vi "MergeFiles.vi"(8 "输出结果":refnum<vi>, 9 "SelectedFormat":refnum<vi>, 10 "FileList":refnum<vi>, 11 "FilesArry":refnum<vi>) -> (2 "Path":path)   [LabVIEW 2015]
panel:
  out "Arry 2":path[](array[path])
  out "第二个子数组":string[](array[string])
  out "Value":string[][](array[string])
  out "Arry1":path[](array[path])
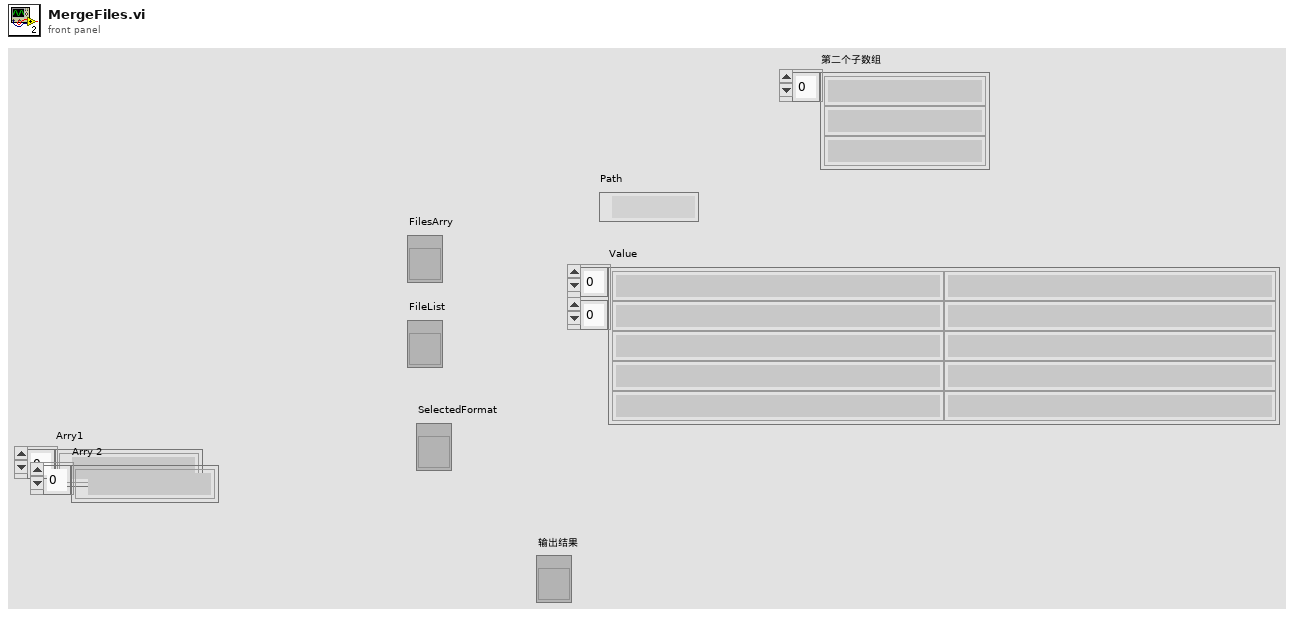
[diagram p1: front panel]
types:
  T1 = enum16{"big-endian, network order", "native, host order", "little-endian"}
  T2 = enum16{"open", "replace", "create", "open or create", "replace or create", "replace or create with confirmation"}
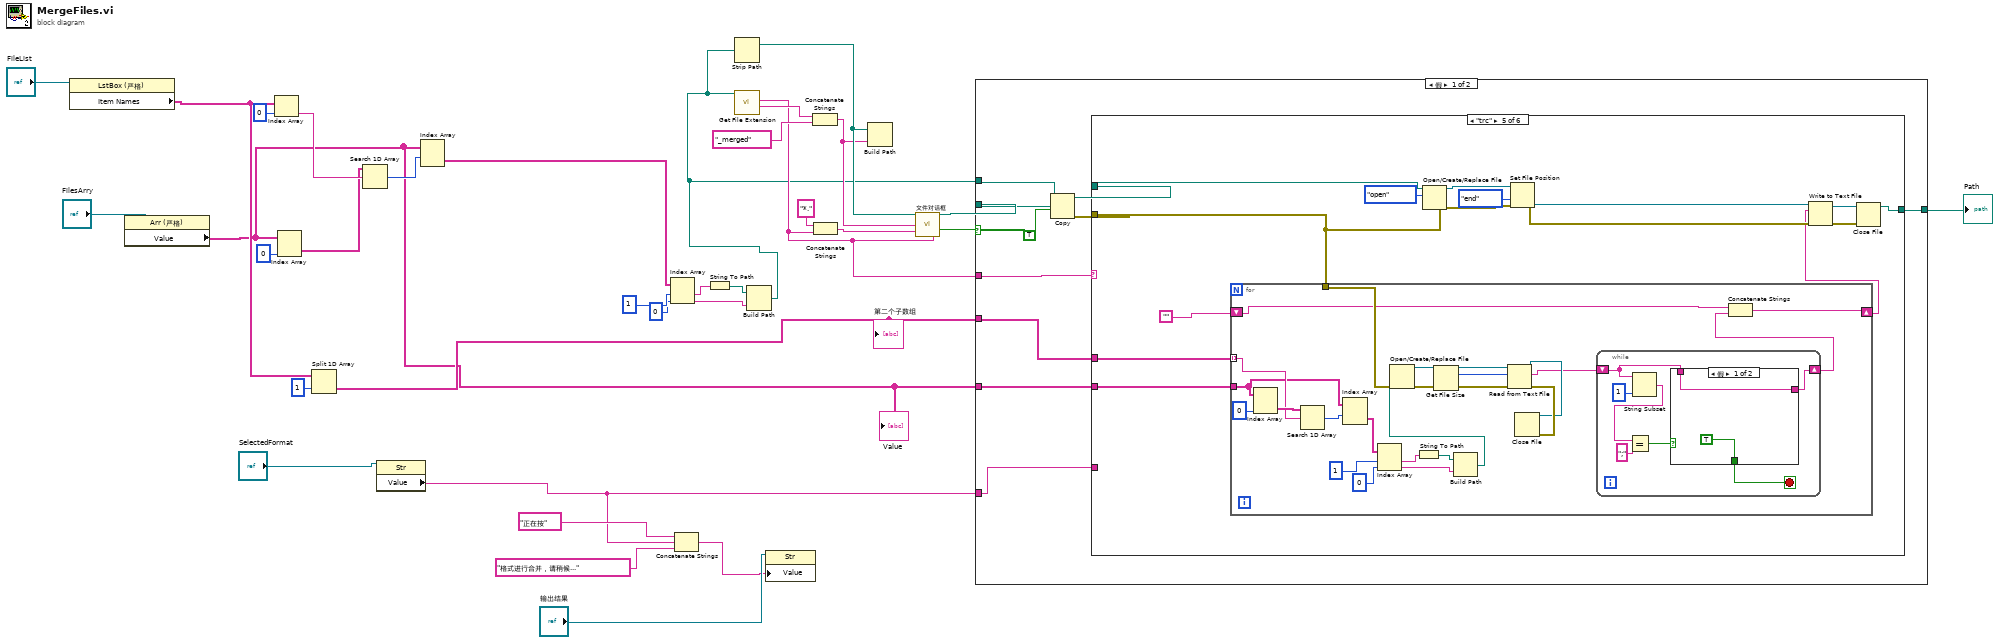
[diagram p0: block diagram]
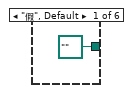
[diagram p2: hidden frame]
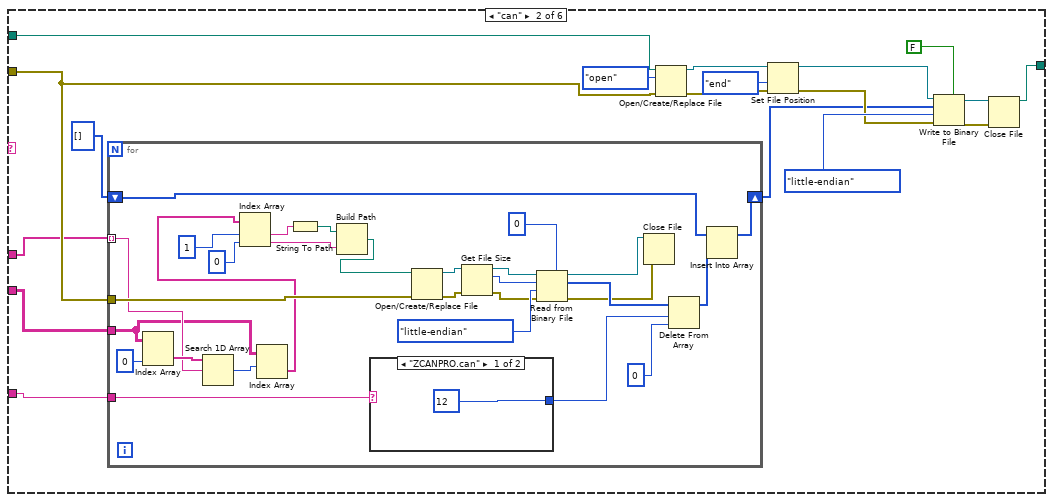
[diagram p3: hidden frame]
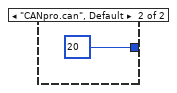
[diagram p4: hidden frame]
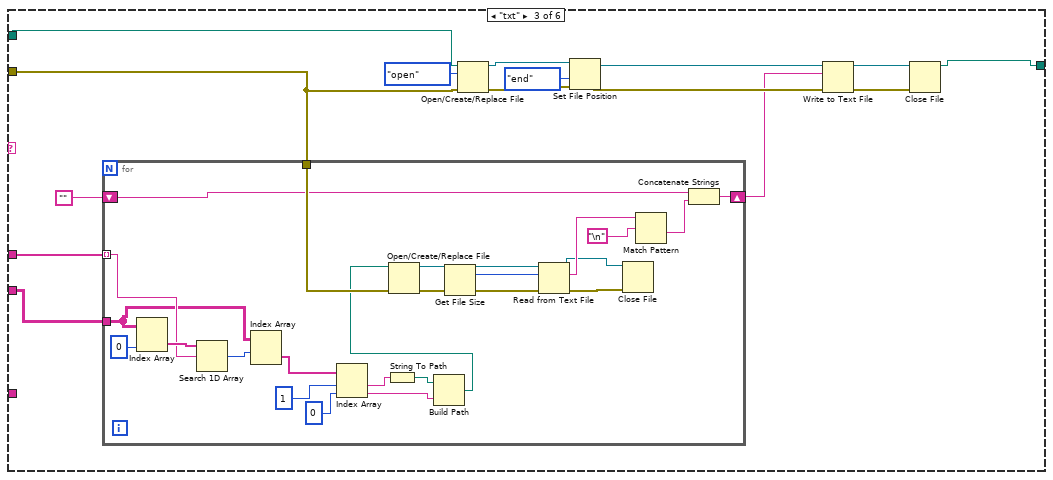
[diagram p5: hidden frame]
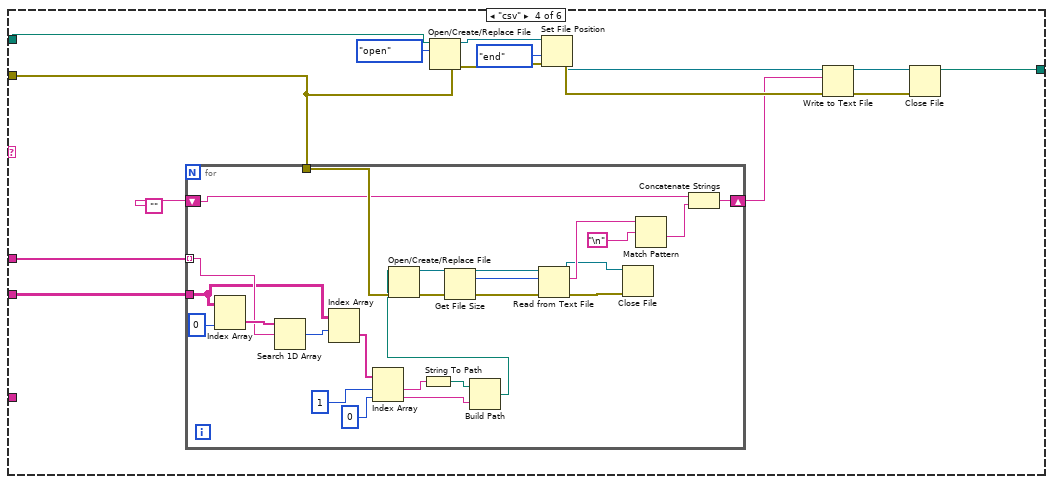
[diagram p6: hidden frame]
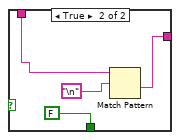
[diagram p7: hidden frame]
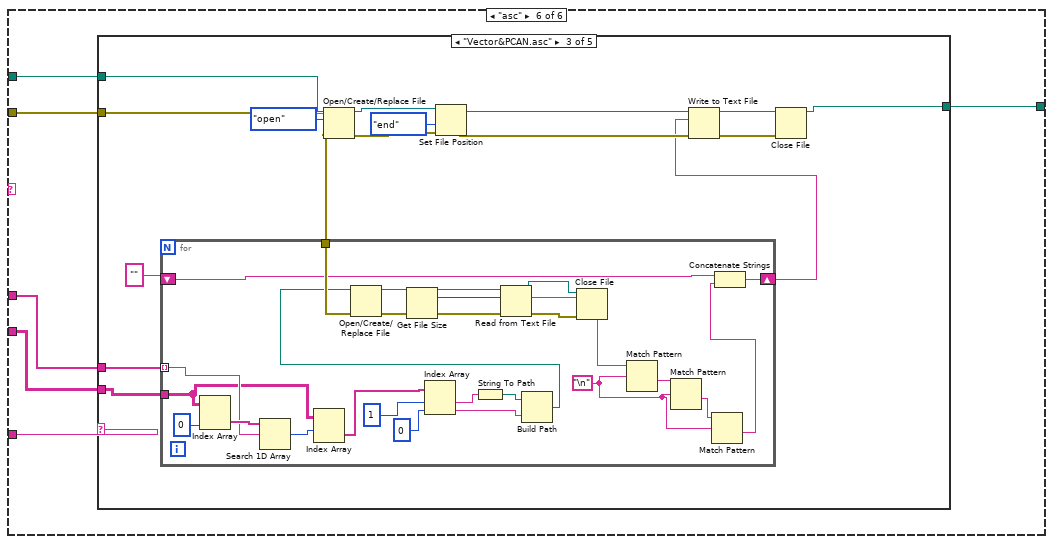
[diagram p8: hidden frame]
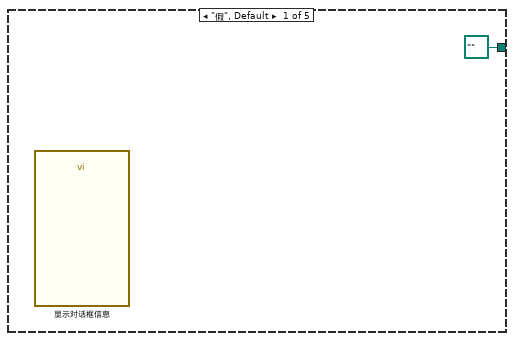
[diagram p9: hidden frame]
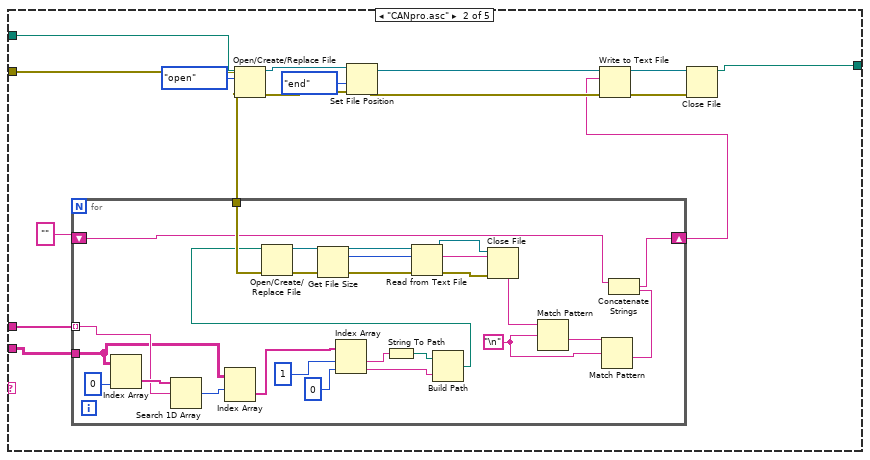
[diagram p10: hidden frame]
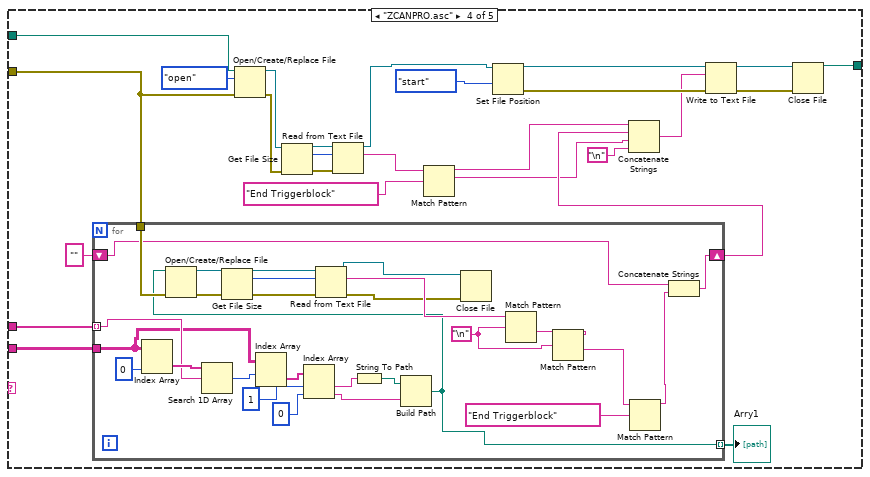
[diagram p11: hidden frame]
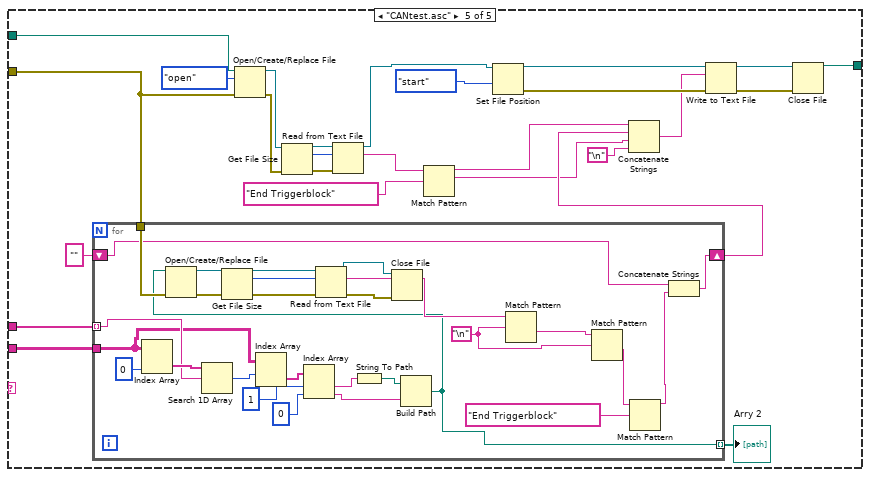
[diagram p12: hidden frame]
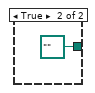
[diagram p13: hidden frame]
diagram:
  n1 = property class="LstBox (严格)"(reference="FileList") -> ("Item Names"=w10:string[])  [unwired: 1 in, 2 out]
  n2 = property class="Arr (严格)"(reference="FilesArry") -> ("Value"=w7:string[][])  [unwired: 1 in, 2 out]
  "Value" <- w7
  n3 = Index Array(array=w10, index=0 ("索引")) -> (element=w14:string)
  n4 = Index Array(array=w7, index (col)=0 ("禁用的索引 (列)")) -> (element=w13:string[])  [unwired: 1 in]
  n5 = Split 1D Array(array=w10, index=1 ("索引")) -> (second subarray=w8:string[])  [unwired: 1 out]
  "第二个子数组" <- w8
  n6 = Search 1D Array(1D array=w13, element=w14) -> (index of element=w12:i32)  [unwired: 1 in]
  n7 = property class="Str"(reference="SelectedFormat") -> ("Value"=w3:string)  [unwired: 1 in, 2 out]
  n8 = Index Array(array=w7, index (row)=w12) -> (element=w11:string[])  [unwired: 1 in]
  n9 = Index Array(array=w11, index #1=1 ("索引"), index #2=0 ("索引")) -> (element #1=w20:string, element #2=w18:string)
  n10 = Concatenate Strings("正在按", w3, "格式进行合并，请稍候...") -> (w1:string)
  n11 = String To Path(string=w20) -> (path=w19:path)
  n12 = Build Path(base path=w19, name or relative path=w18) -> (appended path=w17:path)
  n13 = Strip Path(path=w17) -> (stripped path=w30:path)  [unwired: 1 out]
  n14 = call <vilib>:"Get File Extension.vi"("file"=w17) -> ("filename without extension"=w27:string, "lowercase file extension"=w23:string)  [unwired: 6 in, 3 out]
  n15 = property class="Str"(reference="输出结果", "Value"=w1) -> ()  [unwired: 1 in, 2 out]
  n16 = Concatenate Strings(w27, "_merged" ("字符串")) -> (w29:string)
  n17 = Concatenate Strings("*.", w23) -> (w26:string)
  n18 = Build Path(base path=w30, name or relative path=w29) -> ()  [unwired: 1 out]
  n19 = call "文件对话框"("start path"=w30, "default name"=w29, "pattern (all files)"=w26, "pattern label"=w23) -> ("selected path"=w28:path, "cancelled"=w24:bool)  [unwired: 8 in, 2 out]
  n20 = case shown="假" w24 {
    tunnel: w28 -> [w44 _]
    tunnel: w17 -> [w42 _]
    tunnel: w23 -> [w39 _]
    tunnel: w3 -> [w38 _]
    tunnel: w8 -> [w37 _]
    tunnel: w7 -> [w36 _]
    tunnel: [w35 path "" ("path")] -> w6
    frame False {
      n21 = Copy(9:TRUE, 10:w44, 11:w42) -> (0:w40:errorcluster, 3:w43:path)  [unwired: 2 in, 1 out]
      n22 = case shown="\"trc\"" w39 {
        tunnel: w43 -> [_ w62 w108 w148 w188 w232]
        tunnel: w40 -> [_ w53 w104 w144 w184 w231]
        tunnel: w38 -> [_ w52 _ _ _ w230]
        tunnel: w37 -> [_ w49 w98 w138 w178 w229]
        tunnel: w36 -> [_ w47 w96 w136 w176 w228]
        tunnel: [path "" ("path") w46 w95 w135 w175 w227] -> w35
        frame "假", Default {
        }
        frame "can" {
          n23 = for {
            tunnel: w53 -> [w82]
            tunnel: w52 -> [w81]
            tunnel: w49 -> [w67] mode=indexing
            shift-right: [w71] -> w54
            shift-left: u8[] [] -> [w70]
            tunnel: w47 -> [w66]
            n24 = Index Array(array=w66, index (col)=0 ("禁用的索引 (列)")) -> (element=w69:string[])  [unwired: 1 in]
            n25 = Search 1D Array(1D array=w69, element=w67) -> (index of element=w68:i32)  [unwired: 1 in]
            n26 = Index Array(array=w66, index (row)=w68) -> (element=w65:string[])  [unwired: 1 in]
            n27 = Index Array(array=w65, index #1=1 ("索引"), index #2=0 ("索引")) -> (element #1=w74:string, element #2=w78:string)
            n28 = String To Path(string=w74) -> (path=w75:path)
            n29 = Build Path(base path=w75, name or relative path=w78) -> (appended path=w73:path)
            n30 = case shown="\"ZCANPRO.can\"" w81 {
              tunnel: [12 ("长度") 20 ("长度")] -> w84
              frame "ZCANPRO.can" {
              }
              frame "CANpro.can", Default {
              }
            }
            n31 = Open/Create/Replace File(file path (use dialog)=w73, error in=w82) -> (refnum out=w91:refnum<file>, error out=w90:errorcluster)  [unwired: 4 in, 1 out]
            n32 = Get File Size(file=w91, error in=w90) -> (refnum out=w89:refnum<file>, size (in bytes)=w88:i64, 0:w87:errorcluster)
            n33 = Read from Binary File(5:u8 0, 8:w87, 9:T1."little-endian" ("字节顺序(0:big-endian, network order)"), 10:w88, 11:w89) -> (0:w79:errorcluster, 2:w83:u8[], 3:w80:refnum<file>)  [unwired: 1 in, 1 out]
            n34 = Close File(refnum=w80, error in=w79) -> ()  [unwired: 2 out]
            n35 = Delete From Array(array=w83, length=w84, index=0 ("索引")) -> (array with subset deleted=w72:u8[])  [unwired: 1 out]
            n36 = Insert Into Array(array=w70, new element=w72) -> (w71:u8[])  [unwired: 1 in]
          }
          n37 = Open/Create/Replace File(file path (use dialog)=w62, error in=w53, operation (0:open)=T2."open" ("操作(0:open)")) -> (refnum out=w60:refnum<file>, error out=w59:errorcluster)  [unwired: 3 in, 1 out]
          n38 = Set File Position(refnum=w60, from (0:start)=enum16{"start", "end", "current"}."end" ("自（0:起始）"), error in=w59) -> (refnum out=w57:refnum<file>, error out=w58:errorcluster)  [unwired: 1 in]
          n39 = Write to Binary File(file (use dialog)=w57, data=w54, error in=w58, 5:FALSE ("预置数组或字符串大小？ (T)"), 9:T1."little-endian" ("字节顺序(0:big-endian, network order)")) -> (refnum out=w50:refnum<file>, error out=w51:errorcluster)  [unwired: 1 in, 1 out]
          n40 = Close File(refnum=w50, error in=w51) -> (path=w46:path)  [unwired: 1 out]
        }
        frame "txt" {
          n41 = for {
            tunnel: w104 -> [w132]
            tunnel: w98 -> [w113] mode=indexing
            shift-right: [w118] -> w99
            shift-left: "" -> [w117]
            tunnel: w96 -> [w112]
            n42 = Index Array(array=w112, index (col)=0 ("禁用的索引 (列)")) -> (element=w115:string[])  [unwired: 1 in]
            n43 = Search 1D Array(1D array=w115, element=w113) -> (index of element=w114:i32)  [unwired: 1 in]
            n44 = Index Array(array=w112, index (row)=w114) -> (element=w111:string[])  [unwired: 1 in]
            n45 = Index Array(array=w111, index #1=1 ("索引"), index #2=0 ("索引")) -> (element #1=w121:string, element #2=w124:string)
            n46 = String To Path(string=w121) -> (path=w122:path)
            n47 = Build Path(base path=w122, name or relative path=w124) -> (appended path=w120:path)
            n48 = Open/Create/Replace File(file path (use dialog)=w120, error in=w132) -> (refnum out=w134:refnum<file>, error out=w133:errorcluster)  [unwired: 4 in, 1 out]
            n49 = Get File Size(file=w134, error in=w133) -> (refnum out=w130:refnum<file>, size (in bytes)=w131:i64, 0:w129:errorcluster)
            n50 = Read from Text File(file (use dialog)=w130, count=w131, error in=w129) -> (refnum out=w125:refnum<file>, text=w128:string, error out=w126:errorcluster)  [unwired: 1 in, 1 out]
            n51 = Close File(refnum=w125, error in=w126) -> ()  [unwired: 2 out]
            n52 = Match Pattern(string=w128, regular expression="\n") -> (after substring=w119:string)  [unwired: 1 in, 3 out]
            n53 = Concatenate Strings(w117, w119) -> (w118:string)
          }
          n54 = Open/Create/Replace File(file path (use dialog)=w108, error in=w104, operation (0:open)=T2."open" ("操作(0:open)")) -> (refnum out=w107:refnum<file>, error out=w106:errorcluster)  [unwired: 3 in, 1 out]
          n55 = Set File Position(refnum=w107, from (0:start)=enum16{"start", "end", "current"}."end" ("自（0:起始）"), error in=w106) -> (refnum out=w100:refnum<file>, error out=w103:errorcluster)  [unwired: 1 in]
          n56 = Write to Text File(file (use dialog)=w100, text=w99, error in=w103) -> (refnum out=w101:refnum<file>, error out=w102:errorcluster)  [unwired: 1 in, 1 out]
          n57 = Close File(refnum=w101, error in=w102) -> (path=w95:path)  [unwired: 1 out]
        }
        frame "csv" {
          n58 = for {
            tunnel: w144 -> [w172]
            tunnel: w138 -> [w154] mode=indexing
            shift-right: [w158] -> w139
            shift-left: "" -> [w157]
            tunnel: w136 -> [w152]
            n59 = Index Array(array=w152, index (col)=0 ("禁用的索引 (列)")) -> (element=w155:string[])  [unwired: 1 in]
            n60 = Search 1D Array(1D array=w155, element=w154) -> (index of element=w153:i32)  [unwired: 1 in]
            n61 = Index Array(array=w152, index (row)=w153) -> (element=w151:string[])  [unwired: 1 in]
            n62 = Index Array(array=w151, index #1=1 ("索引"), index #2=0 ("索引")) -> (element #1=w161:string, element #2=w164:string)
            n63 = String To Path(string=w161) -> (path=w162:path)
            n64 = Build Path(base path=w162, name or relative path=w164) -> (appended path=w160:path)
            n65 = Open/Create/Replace File(file path (use dialog)=w160, error in=w172) -> (refnum out=w174:refnum<file>, error out=w173:errorcluster)  [unwired: 4 in, 1 out]
            n66 = Get File Size(file=w174, error in=w173) -> (refnum out=w170:refnum<file>, size (in bytes)=w171:i64, 0:w169:errorcluster)
            n67 = Read from Text File(file (use dialog)=w170, count=w171, error in=w169) -> (refnum out=w165:refnum<file>, text=w168:string, error out=w166:errorcluster)  [unwired: 1 in, 1 out]
            n68 = Close File(refnum=w165, error in=w166) -> ()  [unwired: 2 out]
            n69 = Match Pattern(string=w168, regular expression="\n") -> (after substring=w159:string)  [unwired: 1 in, 3 out]
            n70 = Concatenate Strings(w157, w159) -> (w158:string)
          }
          n71 = Open/Create/Replace File(file path (use dialog)=w148, error in=w144, operation (0:open)=T2."open" ("操作(0:open)")) -> (refnum out=w147:refnum<file>, error out=w146:errorcluster)  [unwired: 3 in, 1 out]
          n72 = Set File Position(refnum=w147, from (0:start)=enum16{"start", "end", "current"}."end" ("自（0:起始）"), error in=w146) -> (refnum out=w140:refnum<file>, error out=w143:errorcluster)  [unwired: 1 in]
          n73 = Write to Text File(file (use dialog)=w140, text=w139, error in=w143) -> (refnum out=w141:refnum<file>, error out=w142:errorcluster)  [unwired: 1 in, 1 out]
          n74 = Close File(refnum=w141, error in=w142) -> (path=w135:path)  [unwired: 1 out]
        }
        frame "trc" {
          n75 = for {
            tunnel: w184 -> [w211]
            tunnel: w178 -> [w196] mode=indexing
            shift-right: [w200] -> w179
            shift-left: "" -> [w199]
            tunnel: w176 -> [w194]
            n76 = Index Array(array=w194, index (col)=0 ("禁用的索引 (列)")) -> (element=w197:string[])  [unwired: 1 in]
            n77 = Search 1D Array(1D array=w197, element=w196) -> (index of element=w195:i32)  [unwired: 1 in]
            n78 = Index Array(array=w194, index (row)=w195) -> (element=w193:string[])  [unwired: 1 in]
            n79 = Index Array(array=w193, index #1=1 ("索引"), index #2=0 ("索引")) -> (element #1=w202:string, element #2=w205:string)
            n80 = String To Path(string=w202) -> (path=w203:path)
            n81 = Build Path(base path=w203, name or relative path=w205) -> (appended path=w201:path)
            n82 = Open/Create/Replace File(file path (use dialog)=w201, error in=w211) -> (refnum out=w213:refnum<file>, error out=w212:errorcluster)  [unwired: 4 in, 1 out]
            n83 = Get File Size(file=w213, error in=w212) -> (refnum out=w209:refnum<file>, size (in bytes)=w210:i64, 0:w208:errorcluster)
            n84 = Read from Text File(file (use dialog)=w209, count=w210, error in=w208) -> (refnum out=w206:refnum<file>, text=w191:string, error out=w207:errorcluster)  [unwired: 1 in, 1 out]
            n85 = Close File(refnum=w206, error in=w207) -> ()  [unwired: 2 out]
            n86 = while {
              shift-right: [w214] -> w190
              shift-left: w191 -> [w215]
              stop <- w216 stop-if-true
              n87 = String Subset(string=w215, length (rest)=1 ("长度（剩余）")) -> (substring=w219:string)  [unwired: 1 in]
              n88 = Equal?(x=w219, y=";") -> (x = y?=w217:bool)
              n89 = case shown="假" w217 {
                tunnel: [TRUE FALSE] -> w216
                tunnel: w215 -> [w221 w224]
                tunnel: [w221 w223] -> w214
                frame False {
                }
                frame True {
                  n90 = Match Pattern(string=w224, regular expression="\n") -> (after substring=w223:string)  [unwired: 1 in, 3 out]
                }
              }
            }
            n91 = Concatenate Strings(w199, w190) -> (w200:string)
          }
          n92 = Open/Create/Replace File(file path (use dialog)=w188, error in=w184, operation (0:open)=T2."open" ("操作(0:open)")) -> (refnum out=w187:refnum<file>, error out=w186:errorcluster)  [unwired: 3 in, 1 out]
          n93 = Set File Position(refnum=w187, from (0:start)=enum16{"start", "end", "current"}."end" ("自（0:起始）"), error in=w186) -> (refnum out=w180:refnum<file>, error out=w183:errorcluster)  [unwired: 1 in]
          n94 = Write to Text File(file (use dialog)=w180, text=w179, error in=w183) -> (refnum out=w181:refnum<file>, error out=w182:errorcluster)  [unwired: 1 in, 1 out]
          n95 = Close File(refnum=w181, error in=w182) -> (path=w175:path)  [unwired: 1 out]
        }
        frame "asc" {
          n96 = case shown="\"Vector&PCAN.asc\"" w230 {
            tunnel: w232 -> [_ w247 w288 w341 w395]
            tunnel: w231 -> [_ w243 w284 w339 w393]
            tunnel: w229 -> [_ w238 w279 w321 w375]
            tunnel: w228 -> [_ w235 w276 w318 w372]
            tunnel: [path "" ("path") w234 w275 w317 w371] -> w227
            frame "假", Default {
              n97 = call "显示对话框信息"() -> ()  [unwired: 10 in, 2 out]
            }
            frame "CANpro.asc" {
              n98 = for {
                tunnel: w243 -> [w272]
                tunnel: w238 -> [w252] mode=indexing
                shift-right: [w258] -> w236
                shift-left: "" -> [w256]
                tunnel: w235 -> [w251]
                w265 = "\n"
                n99 = Index Array(array=w251, index (col)=0 ("禁用的索引 (列)")) -> (element=w254:string[])  [unwired: 1 in]
                n100 = Search 1D Array(1D array=w254, element=w252) -> (index of element=w253:i32)  [unwired: 1 in]
                n101 = Index Array(array=w251, index (row)=w253) -> (element=w250:string[])  [unwired: 1 in]
                n102 = Index Array(array=w250, index #1=1 ("索引"), index #2=0 ("索引")) -> (element #1=w260:string, element #2=w263:string)
                n103 = String To Path(string=w260) -> (path=w261:path)
                n104 = Build Path(base path=w261, name or relative path=w263) -> (appended path=w259:path)
                n105 = Open/Create/Replace File(file path (use dialog)=w259, error in=w272) -> (refnum out=w274:refnum<file>, error out=w273:errorcluster)  [unwired: 4 in, 1 out]
                n106 = Get File Size(file=w274, error in=w273) -> (refnum out=w270:refnum<file>, size (in bytes)=w271:i64, 0:w269:errorcluster)
                n107 = Read from Text File(file (use dialog)=w270, count=w271, error in=w269) -> (refnum out=w266:refnum<file>, text=w268:string, error out=w267:errorcluster)  [unwired: 1 in, 1 out]
                n108 = Close File(refnum=w266, error in=w267) -> ()  [unwired: 2 out]
                n109 = Match Pattern(string=w268, regular expression=w265) -> (after substring=w264:string)  [unwired: 1 in, 3 out]
                n110 = Match Pattern(string=w264, regular expression=w265) -> (after substring=w257:string)  [unwired: 1 in, 3 out]
                n111 = Concatenate Strings(w256, w257) -> (w258:string)
              }
              n112 = Open/Create/Replace File(file path (use dialog)=w247, error in=w243, operation (0:open)=T2."open" ("操作(0:open)")) -> (refnum out=w246:refnum<file>, error out=w245:errorcluster)  [unwired: 3 in, 1 out]
              n113 = Set File Position(refnum=w246, from (0:start)=enum16{"start", "end", "current"}."end" ("自（0:起始）"), error in=w245) -> (refnum out=w239:refnum<file>, error out=w242:errorcluster)  [unwired: 1 in]
              n114 = Write to Text File(file (use dialog)=w239, text=w236, error in=w242) -> (refnum out=w240:refnum<file>, error out=w241:errorcluster)  [unwired: 1 in, 1 out]
              n115 = Close File(refnum=w240, error in=w241) -> (path=w234:path)  [unwired: 1 out]
            }
            frame "Vector&PCAN.asc" {
              n116 = for {
                tunnel: w284 -> [w314]
                tunnel: w279 -> [w296] mode=indexing
                shift-right: [w301] -> w277
                shift-left: "" -> [w300]
                tunnel: w276 -> [w295]
                w290 = "\n"
                n117 = Index Array(array=w295, index (col)=0 ("禁用的索引 (列)")) -> (element=w298:string[])  [unwired: 1 in]
                n118 = Search 1D Array(1D array=w298, element=w296) -> (index of element=w297:i32)  [unwired: 1 in]
                n119 = Index Array(array=w295, index (row)=w297) -> (element=w294:string[])  [unwired: 1 in]
                n120 = Index Array(array=w294, index #1=1 ("索引"), index #2=0 ("索引")) -> (element #1=w303:string, element #2=w306:string)
                n121 = String To Path(string=w303) -> (path=w304:path)
                n122 = Build Path(base path=w304, name or relative path=w306) -> (appended path=w302:path)
                n123 = Open/Create/Replace File(file path (use dialog)=w302, error in=w314) -> (refnum out=w316:refnum<file>, error out=w315:errorcluster)  [unwired: 4 in, 1 out]
                n124 = Get File Size(file=w316, error in=w315) -> (refnum out=w312:refnum<file>, size (in bytes)=w313:i64, 0:w311:errorcluster)
                n125 = Read from Text File(file (use dialog)=w312, count=w313, error in=w311) -> (refnum out=w308:refnum<file>, text=w310:string, error out=w309:errorcluster)  [unwired: 1 in, 1 out]
                n126 = Close File(refnum=w308, error in=w309) -> ()  [unwired: 2 out]
                n127 = Match Pattern(string=w310, regular expression=w290) -> (after substring=w307:string)  [unwired: 1 in, 3 out]
                n128 = Match Pattern(string=w307, regular expression=w290) -> (after substring=w292:string)  [unwired: 1 in, 3 out]
                n129 = Match Pattern(string=w292, regular expression=w290) -> (after substring=w291:string)  [unwired: 1 in, 3 out]
                n130 = Concatenate Strings(w300, w291) -> (w301:string)
              }
              n131 = Open/Create/Replace File(file path (use dialog)=w288, error in=w284, operation (0:open)=T2."open" ("操作(0:open)")) -> (refnum out=w287:refnum<file>, error out=w286:errorcluster)  [unwired: 3 in, 1 out]
              n132 = Set File Position(refnum=w287, from (0:start)=enum16{"start", "end", "current"}."end" ("自（0:起始）"), error in=w286) -> (refnum out=w280:refnum<file>, error out=w283:errorcluster)  [unwired: 1 in]
              n133 = Write to Text File(file (use dialog)=w280, text=w277, error in=w283) -> (refnum out=w281:refnum<file>, error out=w282:errorcluster)  [unwired: 1 in, 1 out]
              n134 = Close File(refnum=w281, error in=w282) -> (path=w275:path)  [unwired: 1 out]
            }
            frame "ZCANPRO.asc" {
              n135 = for {
                tunnel: w339 -> [w368]
                tunnel: w321 -> [w348] mode=indexing
                shift-right: [w355] -> w324
                shift-left: "" -> [w353]
                tunnel: [w352] -> w319 mode=indexing
                tunnel: w318 -> [w347]
                w361 = "\n"
                n136 = Index Array(array=w347, index (col)=0 ("禁用的索引 (列)")) -> (element=w350:string[])  [unwired: 1 in]
                n137 = Search 1D Array(1D array=w350, element=w348) -> (index of element=w349:i32)  [unwired: 1 in]
                n138 = Index Array(array=w347, index (row)=w349) -> (element=w344:string[])  [unwired: 1 in]
                n139 = Index Array(array=w344, index #1=1 ("索引"), index #2=0 ("索引")) -> (element #1=w346:string, element #2=w345:string)
                n140 = String To Path(string=w346) -> (path=w356:path)
                n141 = Build Path(base path=w356, name or relative path=w345) -> (appended path=w352:path)
                n142 = Open/Create/Replace File(file path (use dialog)=w352, error in=w368) -> (refnum out=w370:refnum<file>, error out=w369:errorcluster)  [unwired: 4 in, 1 out]
                n143 = Get File Size(file=w370, error in=w369) -> (refnum out=w366:refnum<file>, size (in bytes)=w367:i64, 0:w365:errorcluster)
                n144 = Read from Text File(file (use dialog)=w366, count=w367, error in=w365) -> (refnum out=w362:refnum<file>, text=w364:string, error out=w363:errorcluster)  [unwired: 1 in, 1 out]
                n145 = Close File(refnum=w362, error in=w363) -> ()  [unwired: 2 out]
                n146 = Match Pattern(string=w364, regular expression=w361) -> (after substring=w360:string)  [unwired: 1 in, 3 out]
                n147 = Match Pattern(string=w360, regular expression=w361) -> (after substring=w358:string)  [unwired: 1 in, 3 out]
                n148 = Match Pattern(string=w358, regular expression="End Triggerblock" ("正则表达式")) -> (before substring=w354:string)  [unwired: 1 in, 3 out]
                n149 = Concatenate Strings(w353, w354) -> (w355:string)
              }
              "Arry1" <- w319
              n150 = Open/Create/Replace File(file path (use dialog)=w341, error in=w339, operation (0:open)=T2."open" ("操作(0:open)")) -> (refnum out=w334:refnum<file>, error out=w333:errorcluster)  [unwired: 3 in, 1 out]
              n151 = Get File Size(file=w334, error in=w333) -> (refnum out=w331:refnum<file>, size (in bytes)=w330:i64, 0:w332:errorcluster)
              n152 = Read from Text File(file (use dialog)=w331, count=w330, error in=w332) -> (refnum out=w328:refnum<file>, text=w329:string)  [unwired: 1 in, 2 out]
              n153 = Match Pattern(string=w329, regular expression="End Triggerblock" ("正则表达式")) -> (before substring=w326:string, match substring=w323:string)  [unwired: 1 in, 2 out]
              n154 = Set File Position(refnum=w328, from (0:start)=enum16{"start", "end", "current"}."start" ("自（0:起始）")) -> (refnum out=w335:refnum<file>, error out=w338:errorcluster)  [unwired: 2 in]
              n155 = Concatenate Strings(w326, w324, w323, "\n") -> (w325:string)
              n156 = Write to Text File(file (use dialog)=w335, text=w325, error in=w338) -> (refnum out=w336:refnum<file>, error out=w337:errorcluster)  [unwired: 1 in, 1 out]
              n157 = Close File(refnum=w336, error in=w337) -> (path=w317:path)  [unwired: 1 out]
            }
            frame "CANtest.asc" {
              n158 = for {
                tunnel: w393 -> [w422]
                tunnel: w375 -> [w402] mode=indexing
                shift-right: [w409] -> w378
                shift-left: "" -> [w407]
                tunnel: [w406] -> w373 mode=indexing
                tunnel: w372 -> [w401]
                w415 = "\n"
                n159 = Index Array(array=w401, index (col)=0 ("禁用的索引 (列)")) -> (element=w404:string[])  [unwired: 1 in]
                n160 = Search 1D Array(1D array=w404, element=w402) -> (index of element=w403:i32)  [unwired: 1 in]
                n161 = Index Array(array=w401, index (row)=w403) -> (element=w398:string[])  [unwired: 1 in]
                n162 = Index Array(array=w398, index #1=1 ("索引"), index #2=0 ("索引")) -> (element #1=w400:string, element #2=w399:string)
                n163 = String To Path(string=w400) -> (path=w410:path)
                n164 = Build Path(base path=w410, name or relative path=w399) -> (appended path=w406:path)
                n165 = Open/Create/Replace File(file path (use dialog)=w406, error in=w422) -> (refnum out=w424:refnum<file>, error out=w423:errorcluster)  [unwired: 4 in, 1 out]
                n166 = Get File Size(file=w424, error in=w423) -> (refnum out=w420:refnum<file>, size (in bytes)=w421:i64, 0:w419:errorcluster)
                n167 = Read from Text File(file (use dialog)=w420, count=w421, error in=w419) -> (refnum out=w416:refnum<file>, text=w418:string, error out=w417:errorcluster)  [unwired: 1 in, 1 out]
                n168 = Close File(refnum=w416, error in=w417) -> ()  [unwired: 2 out]
                n169 = Match Pattern(string=w418, regular expression=w415) -> (after substring=w414:string)  [unwired: 1 in, 3 out]
                n170 = Match Pattern(string=w414, regular expression=w415) -> (after substring=w412:string)  [unwired: 1 in, 3 out]
                n171 = Match Pattern(string=w412, regular expression="End Triggerblock" ("正则表达式")) -> (before substring=w408:string)  [unwired: 1 in, 3 out]
                n172 = Concatenate Strings(w407, w408) -> (w409:string)
              }
              "Arry 2" <- w373
              n173 = Open/Create/Replace File(file path (use dialog)=w395, error in=w393, operation (0:open)=T2."open" ("操作(0:open)")) -> (refnum out=w388:refnum<file>, error out=w387:errorcluster)  [unwired: 3 in, 1 out]
              n174 = Get File Size(file=w388, error in=w387) -> (refnum out=w385:refnum<file>, size (in bytes)=w384:i64, 0:w386:errorcluster)
              n175 = Read from Text File(file (use dialog)=w385, count=w384, error in=w386) -> (refnum out=w382:refnum<file>, text=w383:string)  [unwired: 1 in, 2 out]
              n176 = Match Pattern(string=w383, regular expression="End Triggerblock" ("正则表达式")) -> (before substring=w380:string, match substring=w377:string)  [unwired: 1 in, 2 out]
              n177 = Set File Position(refnum=w382, from (0:start)=enum16{"start", "end", "current"}."start" ("自（0:起始）")) -> (refnum out=w389:refnum<file>, error out=w392:errorcluster)  [unwired: 2 in]
              n178 = Concatenate Strings(w380, w378, w377, "\n") -> (w379:string)
              n179 = Write to Text File(file (use dialog)=w389, text=w379, error in=w392) -> (refnum out=w390:refnum<file>, error out=w391:errorcluster)  [unwired: 1 in, 1 out]
              n180 = Close File(refnum=w390, error in=w391) -> (path=w371:path)  [unwired: 1 out]
            }
          }
        }
      }
    }
    frame True {
    }
  }
  "Path" <- w6
